vi "Destroy.vi"(8 "Error In":errorcluster, 11 "Session":refnum<class "Session.lvclass">) -> (0 "Error Out":errorcluster, 3 "labssh2 Shared Library":path)   [LabVIEW 2017, in "LabSSH2.lvlib" / "Session.lvclass"]
uses:
  Session.lvclass
  Typedefs/Modes.ctl
  Session.lvclass/Session.ctl
  <vilib>/Utility/error.llb/Error Cluster From Error Code.vi
  <vilib>/ErrorRing/Error Ring.xnode
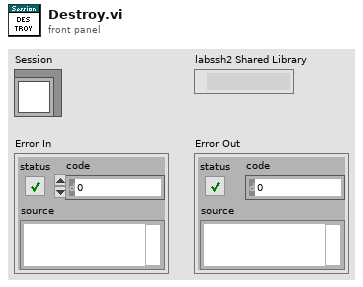
[diagram p1: front panel]
types:
  T1 = typedef "LabSSH2.lvlib/Session.lvclass/Modes.ctl" = enum32{"Non-Blocking", "Blocking"}
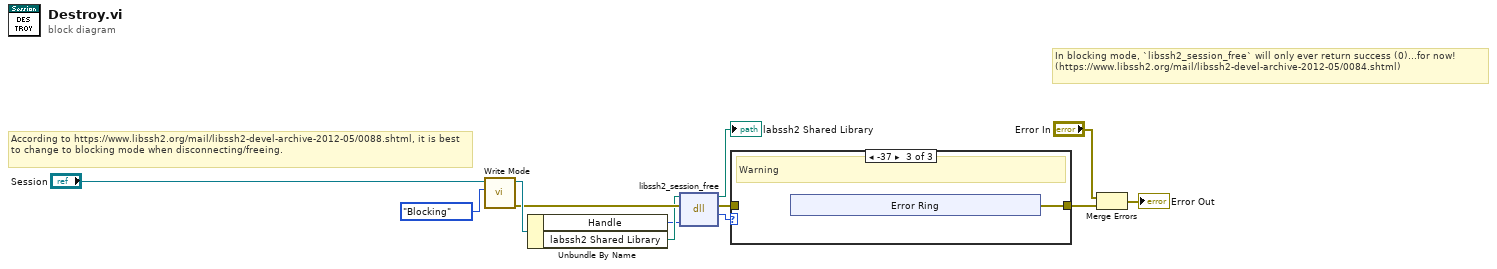
[diagram p0: block diagram]
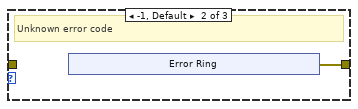
[diagram p3: hidden frame]
diagram:
  # "In blocking mode, `libssh2_session_free` will only ever return success (0)...for now! (https://www.libssh2.org/mail/libssh2-devel-archive-2012-05/0084.shtml)"
  # "According to https://www.libssh2.org/mail/libssh2-devel-archive-2012-05/0088.shtml, it is best to change to blocking mode when disconnecting/freeing."
  n1 = call "Write Mode.vi"("Mode"=Modes."Blocking", "Session In"="Session") -> ("Error Out"=w4:errorcluster, "Sesssion Out"=w5:refnum<class "Session.lvclass">)  [unwired: 8 in]
  n2 = Unbundle By Name(w5) -> ("Handle"=w2:u64, "labssh2 Shared Library"=w3:path)
  n3 = dll-call lib="D:/Users/cfield/Code/Field R&D Services/SSH/LabSSH2/LabVIEW/trunk/src/LabSSH2/Private/labssh2.*" fn="libssh2_session_free"(path in=w3, error in=w4, "session"=w2) -> (path out=→"labssh2 Shared Library":path, error out=w9:errorcluster, "result"=w8:i32)  [unwired: 2 in]
  n4 = case shown="-37" w8 {
    tunnel: w9 -> [w13 _ _]
    tunnel: [w13 w14 w19] -> w7
    frame 0 {
      # "Success"
    }
    frame -1, Default {
      # "Unknown error code"
      n5 = xnode "Error Ring"() -> ("error out"=w14:errorcluster)
    }
    frame -37 {
      # "Warning"
      n6 = xnode "Error Ring"() -> ("error out"=w19:errorcluster)
    }
  }
  n7 = Merge Errors("Error In", w7) -> (→"Error Out":errorcluster)
